vi "DbInterpolation.vi"(9 "Frequency":dbl[](array[numeric]), 11 "Transfers":dbl[](array[numeric])) -> (3 "interpolated val":dbl)   [LabVIEW 2021]
panel:
  out "b":dbl
  out "a":dbl
  out "Y2 flip":dbl
  out "Y1 flip":dbl
  out "X2 flip":dbl
  out "X1 flip":dbl
  out "Selected index":i32
  out "X2":dbl
  out "X1":dbl
  out "Y2":dbl
  out "Y1":dbl
  out "min index(es) 2":i32
  out "abs(x)":dbl[](array[numeric])
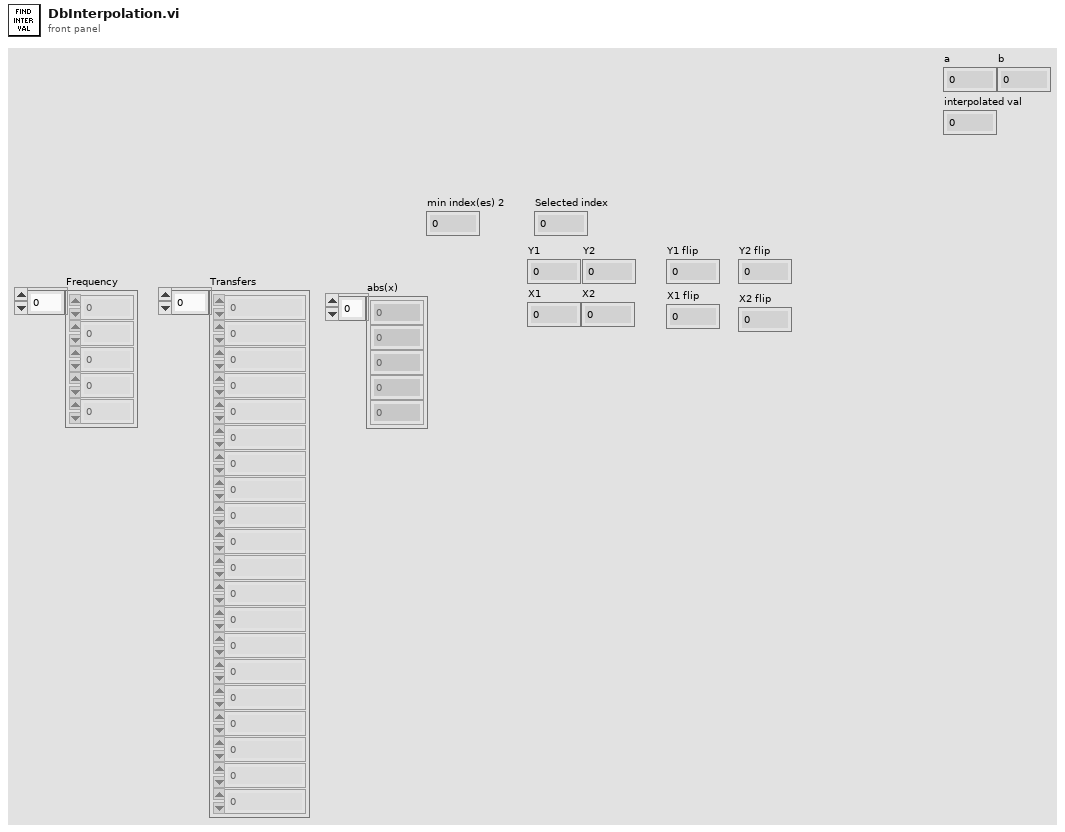
[diagram p1: front panel]
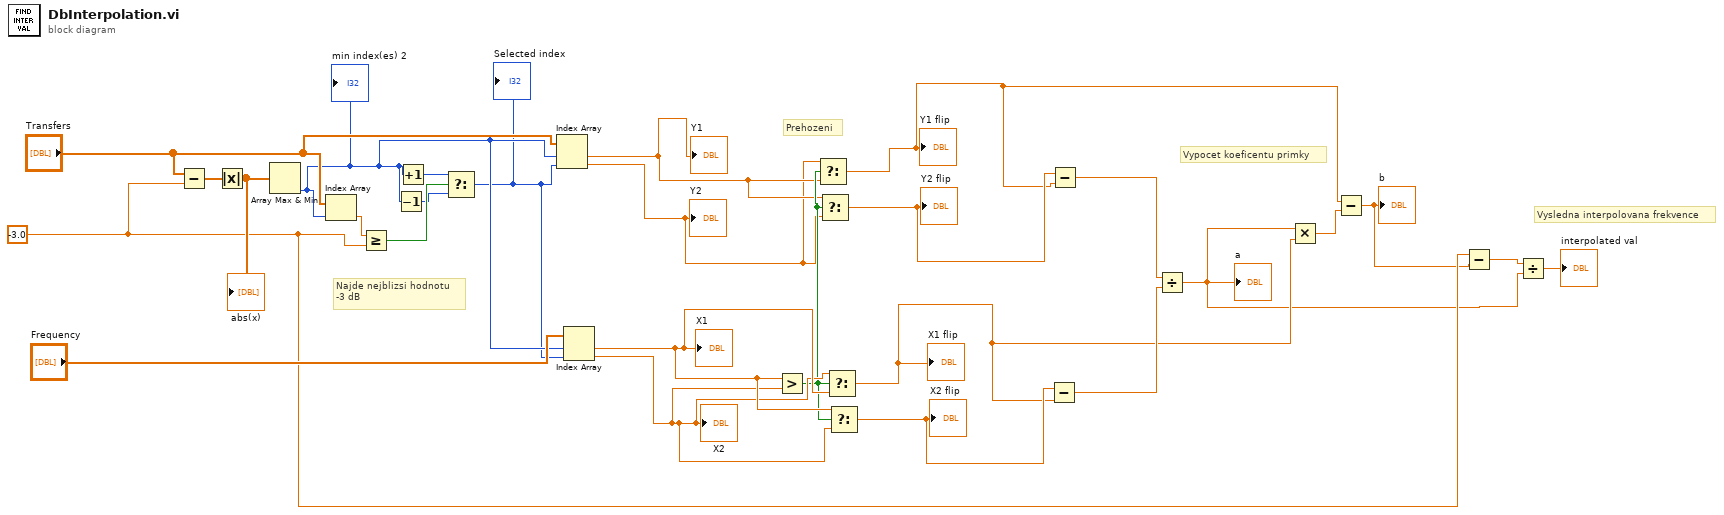
[diagram p0: block diagram]
diagram:
  w5 = -3.0 ("Wanted value")
  # "Vysledna interpolovana frekvence"
  # "Vypocet koeficentu primky"
  # "Prehozeni"
  # "Najde nejblizsi hodnotu \n-3 dB"
  n1 = Subtract(x="Transfers", y=w5) -> (x-y=w27:dbl[])
  n2 = Absolute Value(x=w27) -> (abs(x)=w26:dbl[])
  "abs(x)" <- w26
  n3 = Array Max & Min(array=w26) -> (min index (indices)=w19:i32)  [unwired: 3 out]
  "min index(es) 2" <- w19
  n4 = Index Array(array="Transfers", index=w19) -> (element=w22:dbl)
  n5 = Greater Or Equal?(x=w22, y=w5) -> (x >= y?=w25:bool)
  n6 = Decrement(x=w19) -> (x-1=w23:i32)
  n7 = Increment(x=w19) -> (x+1=w24:i32)
  n8 = Select(t=w24, s=w25, f=w23) -> (s? t:f=w18:i32)
  "Selected index" <- w18
  n9 = Index Array(array="Transfers", index #1=w19, index #2=w18) -> (element #1=w14:dbl, element #2=w13:dbl)
  "Y1" <- w14
  "Y2" <- w13
  n10 = Index Array(array="Frequency", index #1=w19, index #2=w18) -> (element #1=w17:dbl, element #2=w16:dbl)
  "X1" <- w17
  "X2" <- w16
  n11 = Greater?(x=w17, y=w16) -> (0:w15:bool)
  n12 = Select(t=w13, s=w15, f=w14) -> (s? t:f=w6:dbl)
  "Y1 flip" <- w6
  n13 = Select(t=w14, s=w15, f=w13) -> (s? t:f=w12:dbl)
  "Y2 flip" <- w12
  n14 = Select(t=w16, s=w15, f=w17) -> (s? t:f=w8:dbl)
  "X1 flip" <- w8
  n15 = Select(t=w17, s=w15, f=w16) -> (s? t:f=w11:dbl)
  "X2 flip" <- w11
  n16 = Subtract(x=w11, y=w8) -> (x-y=w9:dbl)
  n17 = Subtract(x=w12, y=w6) -> (x-y=w10:dbl)
  n18 = Divide(x=w10, y=w9) -> (x/y=w2:dbl)
  "a" <- w2
  n19 = Multiply(x=w2, y=w8) -> (x*y=w7:dbl)
  n20 = Subtract(x=w6, y=w7) -> (x-y=w4:dbl)
  "b" <- w4
  n21 = Subtract(x=w5, y=w4) -> (x-y=w3:dbl)
  n22 = Divide(x=w3, y=w2) -> (x/y=→"interpolated val":dbl)
